vi "getVoltagesamples.vi"(8 "error in (no error)":errorcluster, 11 "params":refnum<class "JSON Value.lvclass">) -> (0 "error out":errorcluster, 3 "data":refnum<class "JSON Value.lvclass">)   [LabVIEW 2017]
uses:
  <vilib>/NI/JSON Support for LabVIEW/JSON Value/JSON Value.lvclass
  <vilib>/DAQmx/read.llb/DAQmx Read (Analog 1D DBL 1Chan NSamp).vi
  <vilib>/NI/JSON Support for LabVIEW/JSON Value/Object/Get Value/Get Value (Numeric).vi
  <vilib>/NI/JSON Support for LabVIEW/JSON Value/Object/Get Value/Get Value (String).vi
  <vilib>/DAQmx/create/channels.llb/DAQmx Create Channel (AI-Voltage-Basic).vi
  <vilib>/DAQmx/configure/timing.llb/DAQmx Timing (Sample Clock).vi
  <vilib>/DAQmx/miscellaneous.llb/DAQmx Fill In Error Info.vi
  <vilib>/NI/JSON Support for LabVIEW/JSON Value/New JSON Value/New JSON (Numeric[]).vi
  <vilib>/NI/JSON Support for LabVIEW/JSON Value/New JSON Value/New JSON (Numeric).vi
  <vilib>/NI/JSON Support for LabVIEW/JSON Value/New JSON Value/New JSON ({Value[]}).vi
  <vilib>/NI/NI JSONRPC Server Framework/Classes/Server/JSONRPC Server.lvclass
  <resource>/objmgr/daqmx.rc
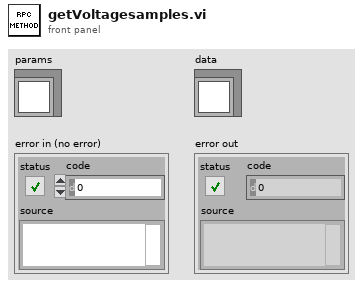
[diagram p1: front panel]
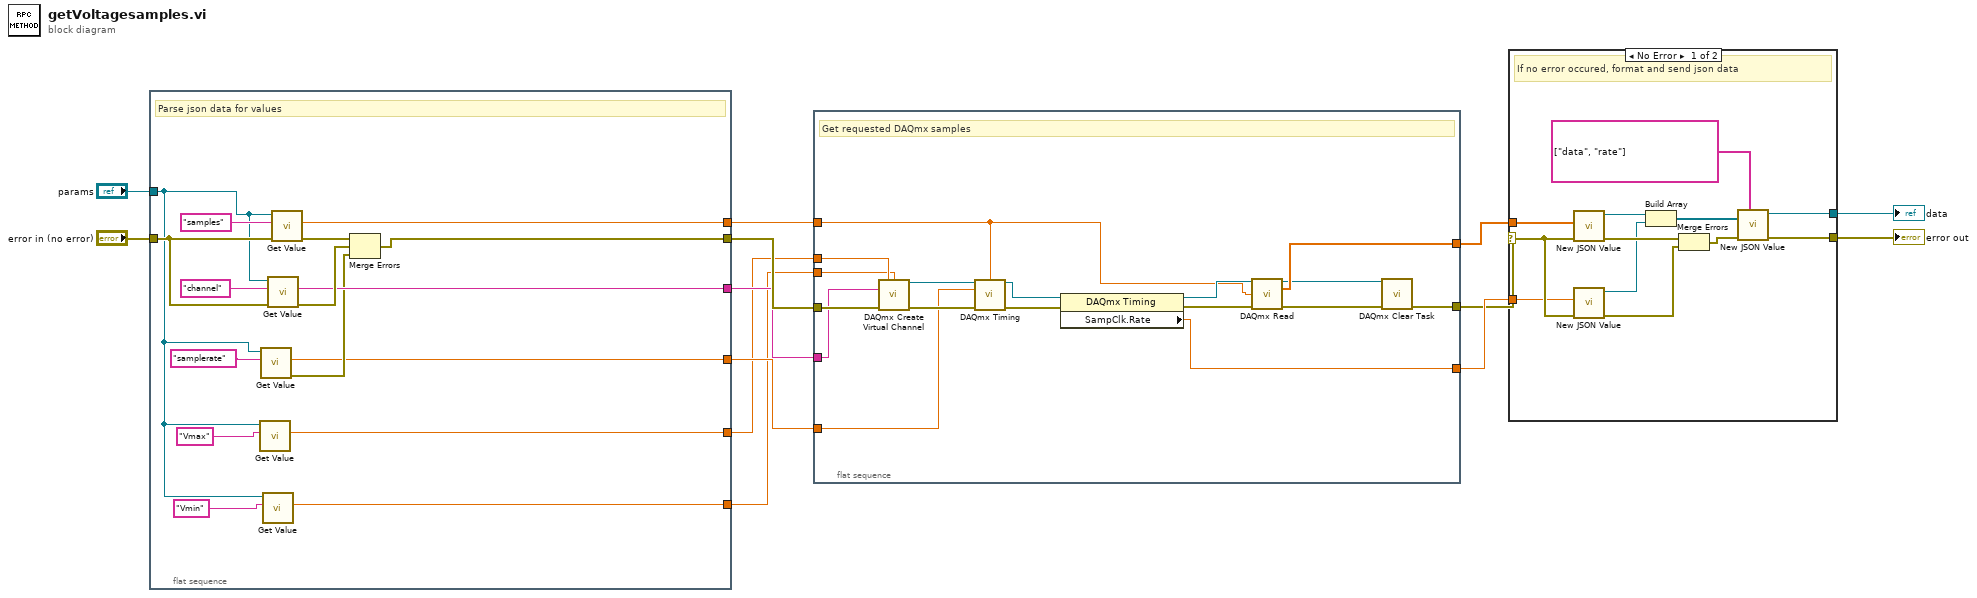
[diagram p0: block diagram]
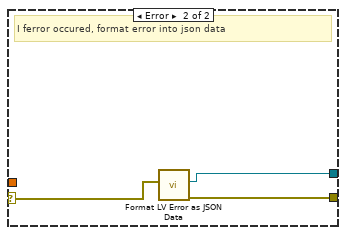
[diagram p2: hidden frame]
diagram:
  n1 = flat-sequence {
    tunnel: "params" -> [w18]
    tunnel: "error in (no error)" -> [w22]
    tunnel: [w26] -> w11
    tunnel: [w24] -> w5
    tunnel: [w23] -> w6
    tunnel: [w19] -> w3
    tunnel: [w15] -> w2
    tunnel: [w14] -> w1
    frame #0 {
      # "Parse json data for values"
      n2 = call-poly <vilib>:"Get Value.vi"("key"="Vmax", "JSON Value in"=w18) -> ("value"=w15:dbl)  [unwired: 8 in, 1 out]
      n3 = call-poly <vilib>:"Get Value.vi"("key"="samplerate", "JSON Value in"=w18) -> ("error out"=w20:errorcluster, "value"=w19:dbl)  [unwired: 8 in]
      n4 = call-poly <vilib>:"Get Value.vi"("key"="Vmin", "JSON Value in"=w18) -> ("value"=w14:dbl)  [unwired: 8 in, 1 out]
      n5 = call-poly <vilib>:"Get Value.vi"("error in (no error)"=w22, "key"="channel", "JSON Value in"=w18) -> ("error out"=w25:errorcluster, "value"=w23:string)  [unwired: 7 in]
      n6 = call-poly <vilib>:"Get Value.vi"("error in (no error)"=w22, "key"="samples", "JSON Value in"=w18) -> ("error out"=w27:errorcluster, "value"=w24:dbl)  [unwired: 7 in]
      n7 = Merge Errors(w27, w25, w20) -> (w26:errorcluster)
    }
  }
  n8 = flat-sequence {
    tunnel: w11 -> [w46]
    tunnel: [w40] -> w8
    tunnel: [w36] -> w7
    tunnel: w6 -> [w45]
    tunnel: w5 -> [w37]
    tunnel: [w33] -> w4
    tunnel: w3 -> [w32]
    tunnel: w2 -> [w31]
    tunnel: w1 -> [w30]
    frame #0 {
      # "Get requested DAQmx samples"
      n9 = call-poly <vilib>:"DAQmx Create Virtual Channel.vi"("maximum value"=w31, "minimum value"=w30, "physical channels"=w45, "error in"=w46) -> ("task out"=w43:refnum<k21>, "error out"=w44:errorcluster)  [unwired: 10 in]
      n10 = call-poly <vilib>:"DAQmx Timing.vi"("task/channels in"=w43, "samples per channel"=w37, "rate"=w32, "error in"=w44) -> ("task out"=w41:refnum<k21>, "error out"=w42:errorcluster)  [unwired: 10 in]
      n11 = property class="DAQmx Timing"(reference=w41, error in=w42) -> (reference out=w38:refnum<k21>, error out=w39:errorcluster, "SampClk.Rate"=w40:dbl)
      n12 = call-poly <vilib>:"DAQmx Read.vi"("task/channels in"=w38, "number of samples per channel"=w37, "error in"=w39) -> ("task out"=w34:refnum<k21>, "data"=w36:dbl[], "error out"=w35:errorcluster)  [unwired: 10 in]
      n13 = call <vilib>:"DAQmx Clear Task.vi"("task in"=w34, "error in"=w35) -> ("error out"=w33:errorcluster)  [unwired: 13 in]
    }
  }
  n14 = case shown="No Error" w4 {
    selector: w4 -> [w52 w61]
    tunnel: [w57 w59] -> w10
    tunnel: [w51 w60] -> w9
    tunnel: w7 -> [w50 _]
    tunnel: w8 -> [w47 _]
    frame No Error {
      # "If no error occured, format and send json data"
      n15 = call-poly <vilib>:"New JSON Value.vi"("error in (no error)"=w52, "Numeric Array"=w50) -> ("error out"=w58:errorcluster, "JSON Value out"=w56:refnum<class "JSON Value.lvclass">)  [unwired: 8 in]
      n16 = call-poly <vilib>:"New JSON Value.vi"("error in (no error)"=w52, "value"=w47) -> ("error out"=w53:errorcluster, "JSON Value out"=w55:refnum<class "JSON Value.lvclass">)  [unwired: 8 in]
      n17 = Build Array(w56, w55) -> (w49:refnum<class "JSON Value.lvclass">[])
      n18 = Merge Errors(w58, w53) -> (w54:errorcluster)
      n19 = call-poly <vilib>:"New JSON Value.vi"("keys"=string[] ["data", "rate"], "error in (no error)"=w54, "values"=w49) -> ("error out"=w57:errorcluster, "JSON Value out"=w51:refnum<class "JSON Value.lvclass">)  [unwired: 7 in]
    }
    frame Error {
      # "I ferror occured, format error into json data"
      n20 = call <vilib>:"Format LV Error as JSON Data.vi"("error in"=w61) -> ("error out"=w59:errorcluster, "Error Value out"=w60:refnum<class "JSON Value.lvclass">)  [unwired: 9 in]
    }
  }
  "data" <- w9
  "error out" <- w10
